vi "Configure Dialog.vi"(8 "error in (no error)":errorcluster, 11 "Configure Edge Trigger Source Msg.lvclass":refnum<class "Configure Edge Trigger Source Msg.lvclass">) -> (0 "error out":errorcluster, 2 "Ok?":bool, 3 "Configure Edge Trigger Source Msg.lvclass":refnum<class "Configure Edge Trigger Source Msg.lvclass">)   [LabVIEW 2014, in "CS++Scope.lvlib" / "Configure Edge Trigger Source Msg.lvclass"]
uses:
  Configure Edge Trigger Source Msg.lvclass
  Configure Edge Trigger Source Msg.lvclass/Configure Edge Trigger Source Msg.ctl
panel:
  in  "trigger slope (Positive)":i32(ring)=1 items=["Positive"=1, "Negative"=0]
  in  "trigger level  (0.0 V)":dbl[unit]
  in  "trigger source (CHANNEL1)":string
  in  "Cancel Button":bool
  in  "OK Button":bool
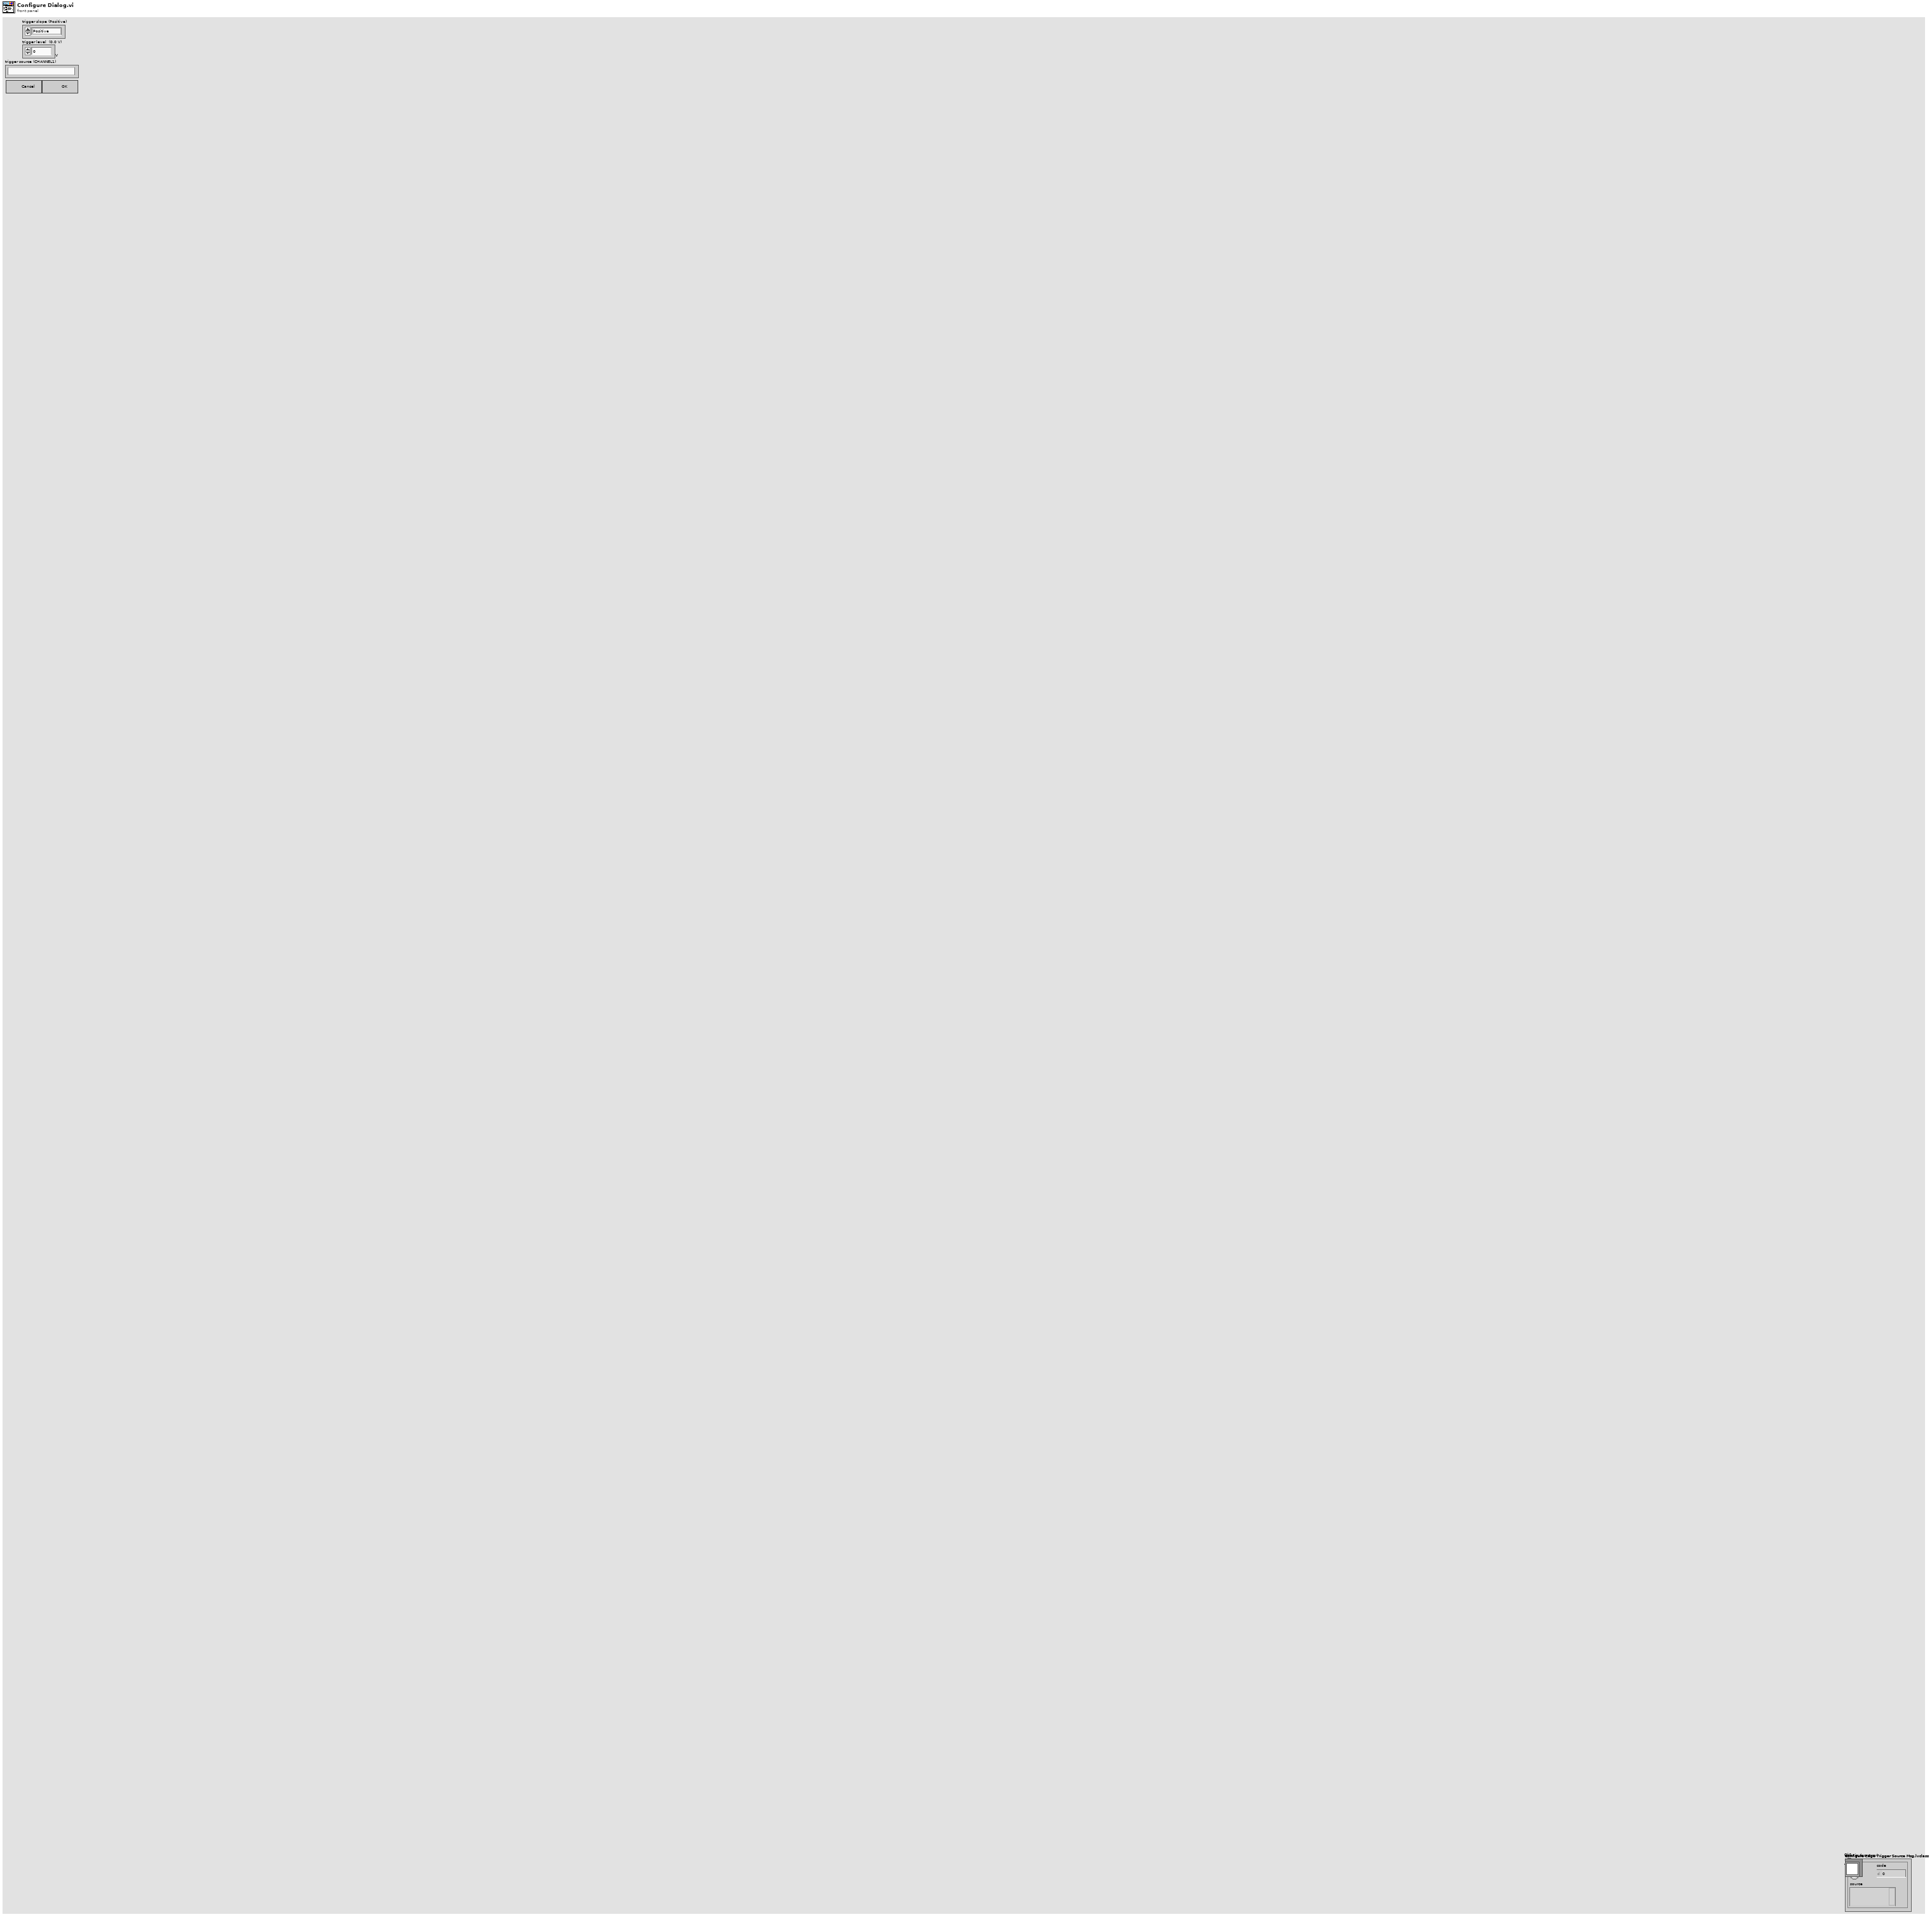
[diagram p1: front panel]
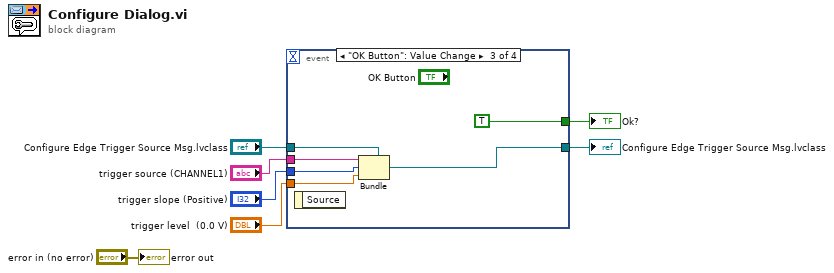
[diagram p0: block diagram]
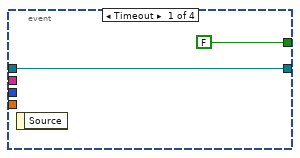
[diagram p2: hidden frame]
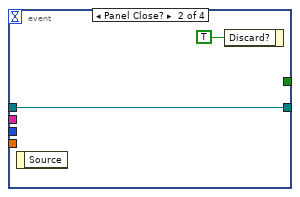
[diagram p3: hidden frame]
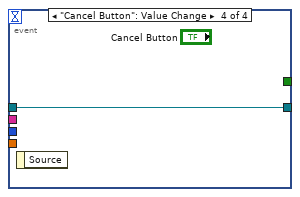
[diagram p4: hidden frame]
diagram:
  n1 = event shown="[2] \"OK Button\": Value Change" {
    selector: _ -> [_ _ _ _]
    dyn-events: _ -> [_ _ _ _]
    timeout: _ -> [_ _ _ _]
    tunnel: [w8 w10 w15 w18] -> w5
    tunnel: "Configure Edge Trigger Source Msg.lvclass" -> [w8 w10 w17 w18]
    tunnel: [FALSE _ TRUE _] -> w6
    tunnel: "trigger source (CHANNEL1)" -> [_ _ w14 _]
    tunnel: "trigger slope (Positive)" -> [_ _ w13 _]
    tunnel: "trigger level  (0.0 V)" -> [_ _ w12 _]
    event Timeout {
      n2 = event-data() -> ()  [unwired: 1 in, 1 out]
    }
    event Panel Close? {
      n3 = event-data() -> ()  [unwired: 1 in, 1 out]
      n4 = event-data ("Event Filter Node")("Discard?"=TRUE) -> ()  [unwired: 1 in, 1 out]
    }
    event "OK Button": Value Change {
      n5 = event-data() -> ()  [unwired: 1 in, 1 out]
      n6 = Bundle ("Main-Bundler")(cluster=w17, w14, w13, w12) -> (w15:refnum<class "Configure Edge Trigger Source Msg.lvclass">)
    }
    event "Cancel Button": Value Change {
      n7 = event-data() -> ()  [unwired: 1 in, 1 out]
    }
  }
  "Ok?" <- w6
  "Configure Edge Trigger Source Msg.lvclass" <- w5
  "error out" <- "error in (no error)"
